vi "setUp.vi"(8 "error in":errorcluster, 11 "reference in":refnum<class "Logging Loopback.lvclass">) -> (0 "error out":errorcluster, 3 "reference out":refnum<class "Logging Loopback.lvclass">)   [LabVIEW 2020, in "Logging Loopback.lvclass"]
doc: "setUp runs prior to the test method during test execution. Use this method to initialize any object data required by your tests."
uses:
  Logging Loopback.lvclass
  <vilib>/addons/_JKI Toolkits/VI Tester/TestCase.llb/TestCase.lvclass
  niveristand-custom-device-testing-tools/VeriStandTestUtilities/VeriStandTestUtilities.lvlib
  <vilib>/WebDAVClient/NI_WebDAV.lvlib
  C:/Users/nitest/Desktop/Git 2020/niveristand-custom-device-testing-tools/VeriStandTestCase/VeriStandTestCase.lvclass
  C:/Program Files (x86)/National Instruments/LabVIEW 2020/vi.lib/addons/_JKI Toolkits/VI Tester/TestCase.llb/TestCase.lvclass
  C:/Users/nitest/Desktop/Git 2020/niveristand-ballard-arinc429-custom-device/Source/Custom Device Support/Tests/System/Logging Loopback/Logging Loopback.lvclass
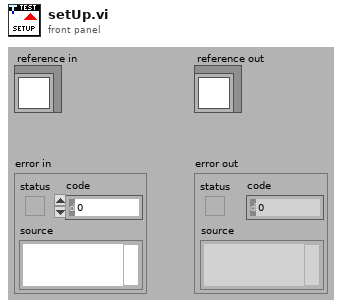
[diagram p1: front panel]
types:
  T1 = typedef "Custom Device API.lvlib/Custom Device Item Ref.ctl" = u64
  T2 = typedef "NI_WebDAV.lvlib/SessionHandle.ctl" = refnum<k1>
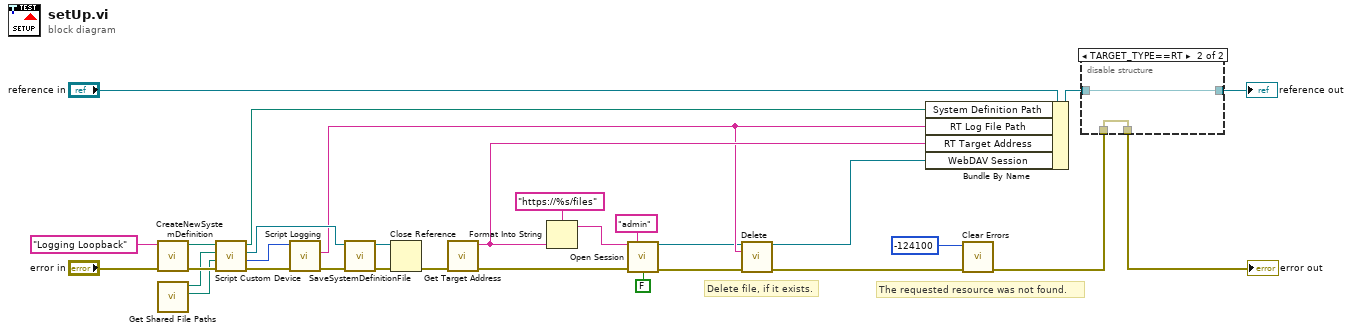
[diagram p0: block diagram]
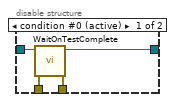
[diagram p2: hidden frame]
diagram:
  # "Delete file, if it exists."
  # "The requested resource was not found."
  n1 = call "CreateNewSystemDefinition.vi"("error in"="error in", "System Definition Name"="Logging Loopback" ("Channel")) -> ("error out"=w27:errorcluster, "System Definition Path"=w26:path)  [unwired: 8 in]
  n2 = call "Get Shared File Paths.vi"() -> ("Hardware File"=w1:path, "Parameters File"=w2:path)  [unwired: 10 in]
  n3 = call "Script Custom Device.vi"("error in"=w27, "Hardware Configuration File Path"=w1, "Parameters Configuration File Path"=w2, "System Definition File Path In"=w26) -> ("error out"=w23:errorcluster, "Ballard ARINC 429 custom device out"=w22:T1, "System Definition Reference"=w25:refnum<k24>, "System Definition File Path Out"=w11:path)  [unwired: 4 in]
  n4 = call "Script Logging.vi"("error in (no error)"=w23, "Ballard ARINC 429 custom device in"=w22) -> ("error out"=w21:errorcluster, "RT log file path"=w14:string)  [unwired: 7 in, 1 out]
  n5 = call "SaveSystemDefinitionFile.vi"("error in (no error)"=w21, "System Definition Reference in"=w25) -> ("error out"=w20:errorcluster, "System Definition Reference out"=w19:refnum<k24>)  [unwired: 8 in]
  n6 = Close Reference(reference=w19, error in (no error)=w20) -> (error out=w17:errorcluster)
  n7 = call "Get Target Address.vi"("error in (no error)"=w17) -> ("error out"=w16:errorcluster, "target address"=w15:string)  [unwired: 9 in]
  n8 = Format Into String(format string="https://%s/files" ("host uri prefix"), w15) -> (resulting string=w4:string)  [unwired: 2 in, 1 out]
  n9 = call <vilib>:"Open Session.vi"("host uri prefix"=w4, "username"="admin", "error in (no error)"=w16, "verify server?"=FALSE) -> ("session handle out"=w8:T2, "error out"=w7:errorcluster)  [unwired: 10 in]
  n10 = call <vilib>:"Delete.vi"("session handle"=w8, "relative uri"=w14, "error in (no error)"=w7) -> ("session handle out"=w9:T2, "error out"=w13:errorcluster)  [unwired: 11 in]
  n11 = Bundle By Name(cluster="reference in", "System Definition Path"=w11, "RT Log File Path"=w14, "RT Target Address"=w15, "WebDAV Session"=w9) -> (w18:refnum<class "Logging Loopback.lvclass">)
  n12 = call <vilib>:"Clear Errors.vi"("error in (no error)"=w13, "specific error code to clear (0: all)"=-124100) -> ("error out"=w10:errorcluster)  [unwired: 4 in, 1 out]
  n13 = disable-structure shown="TARGET_TYPE==RT" {
    disable-tunnel: w10 -> [w35 w36]
    disable-tunnel: [w34 w36] -> w31
    disable-tunnel: [w33 w37] -> w29
    disable-tunnel: w18 -> [w32 w37]
    frame condition #0 (active) {
      n14 = call <vilib>:"WaitOnTestComplete.vi"("error in (no error)"=w35, "TestCase in"=w32) -> ("error out"=w34:errorcluster, "TestCase out"=w33:refnum<class "Logging Loopback.lvclass">)  [unwired: 8 in]
    }
    frame condition #1 {
    }
  }
  "error out" <- w31
  "reference out" <- w29
